vi "example_02_convert.vi"() -> ()   [LabVIEW 2015, in "lv-unit-conversion.lvlib"] (continued)
{"symbol"="bar/h", "name"="bar per hour", "dimension"="M/LT3", "is_si_unit"=TRUE, "category"="derived", "base_unit"="Pa/s", "conversion_reference"="DERIVED", "is_exact"=TRUE, "a"=0.0, "b"=100000.0, "c"=3600.0, "d"=0.0, "underlying_def"="", "description"=""}, {"symbol"="kPa/h", "name"="kilopascal per hour", "dimension"="M/LT3", "is_si_unit"=TRUE, "category"="derived", "base_unit"="Pa/s", "conversion_reference"="DERIVED", "is_exact"=TRUE, "a"=0.0, "b"=1000.0, "c"=3600.0, "d"=0.0, "underlying_def"="", "description"=""}, {"symbol"="kPa/min", "name"="kilopascal per min", "dimension"="M/LT3", "is_si_unit"=TRUE, "category"="derived", "base_unit"="Pa/s", "conversion_reference"="DERIVED", "is_exact"=TRUE, "a"=0.0, "b"=1000.0, "c"=60.0, "d"=0.0, "underlying_def"="", "description"=""}, {"symbol"="MPa/h", "name"="megapascal per hour", "dimension"="M/LT3", "is_si_unit"=TRUE, "category"="derived", "base_unit"="Pa/s", "conversion_reference"="DERIVED", "is_exact"=TRUE, "a"=0.0, "b"=1000000.0, "c"=3600.0, "d"=0.0, "underlying_def"="", "description"=""}, {"symbol"="Pa/h", "name"="pascal per hour", "dimension"="M/LT3", "is_si_unit"=TRUE, "category"="derived", "base_unit"="Pa/s", "conversion_reference"="DERIVED", "is_exact"=TRUE, "a"=0.0, "b"=1.0, "c"=3600.0, "d"=0.0, "underlying_def"="", "description"=""}, {"symbol"="psi/h", "name"="psi per hour", "dimension"="M/LT3", "is_si_unit"=TRUE, "category"="derived", "base_unit"="Pa/s", "conversion_reference"="DERIVED", "is_exact"=TRUE, "a"=0.0, "b"=4.4482216152605, "c"=2.322576, "d"=0.0, "underlying_def"="", "description"=""}, {"symbol"="psi/min", "name"="psi per minute", "dimension"="M/LT3", "is_si_unit"=TRUE, "category"="derived", "base_unit"="Pa/s", "conversion_reference"="DERIVED", "is_exact"=TRUE, "a"=0.0, "b"=4.4482216152605, "c"=0.0387096, "d"=0.0, "underlying_def"="", "description"=""}, {"symbol"="0.001 kPa2/cP", "name"="kilopascal squared per thousand centipoise", "dimension"="M/LT3", "is_si_unit"=TRUE, "category"="derived", "base_unit"="Pa2/(Pa.s)", "conversion_reference"="DERIVED", "is_exact"=TRUE, "a"=0.0, "b"=1000000.0, "c"=1.0, "d"=0.0, "underlying_def"="", "description"=""}, {"symbol"="bar2/cP", "name"="bar squared per centipoise", "dimension"="M/LT3", "is_si_unit"=TRUE, "category"="derived", "base_unit"="Pa2/(Pa.s)", "conversion_reference"="DERIVED", "is_exact"=TRUE, "a"=0.0, "b"=10000000000000.0, "c"=1.0, "d"=0.0, "underlying_def"="", "description"=""}, {"symbol"="kPa2/cP", "name"="kilopascal squared per centipoise", "dimension"="M/LT3", "is_si_unit"=TRUE, "category"="derived", "base_unit"="Pa2/(Pa.s)", "conversion_reference"="DERIVED", "is_exact"=TRUE, "a"=0.0, "b"=1000000000.0, "c"=1.0, "d"=0.0, "underlying_def"="", "description"=""}, {"symbol"="psi2/cP", "name"="psi squared per centipoise", "dimension"="M/LT3", "is_si_unit"=TRUE, "category"="derived", "base_unit"="Pa2/(Pa.s)", "conversion_reference"="DERIVED", "is_exact"=TRUE, "a"=0.0, "b"=19.786675538470732, "c"=4.162314256e-10, "d"=0.0, "underlying_def"="", "description"=""}, {"symbol"="Btu[IT]/(h.ft3)", "name"="BTU per hour cubic foot", "dimension"="M/LT3", "is_si_unit"=TRUE, "category"="derived", "base_unit"="W/m3", "conversion_reference"="DERIVED", "is_exact"=TRUE, "a"=0.0, "b"=1055.05585262, "c"=101.9406477312, "d"=0.0, "underlying_def"="", "description"=""}, {"symbol"="Btu[IT]/(s.ft3)", "name"="(BTU per second) per cubic foot", "dimension"="M/LT3", "is_si_unit"=TRUE, "category"="derived", "base_unit"="W/m3", "conversion_reference"="DERIVED", "is_exact"=TRUE, "a"=0.0, "b"=1055.05585262, "c"=0.028316846592, "d"=0.0, "underlying_def"="", "description"=""}, {"symbol"="cal[th]/(h.cm3)", "name"="calorie per hour cubic centimetre", "dimension"="M/LT3", "is_si_unit"=TRUE, "category"="derived", "base_unit"="W/m3", "conversion_reference"="DERIVED", "is_exact"=TRUE, "a"=0.0, "b"=4.184, "c"=0.0036, "d"=0.0, "underlying_def"="", "description"=""}, {"symbol"="cal[th]/(s.cm3)", "name"="calorie per second cubic centimetre", "dimension"="M/LT3", "is_si_unit"=TRUE, "category"="derived", "base_unit"="W/m3", "conversion_reference"="DERIVED", "is_exact"=TRUE, "a"=0.0, "b"=4184000.0, "c"=1.0, "d"=0.0, "underlying_def"="", "description"=""}, {"symbol"="hp/ft3", "name"="horsepower per cubic foot", "dimension"="M/LT3", "is_si_unit"=TRUE, "category"="derived", "base_unit"="W/m3", "conversion_reference"="DERIVED", "is_exact"=TRUE, "a"=0.0, "b"=745.6998715822702, "c"=0.028316846592, "d"=0.0, "underlying_def"="", "description"=""}, {"symbol"="kW/m3", "name"="kilowatt per cubic metre", "dimension"="M/LT3", "is_si_unit"=TRUE, "category"="derived", "base_unit"="W/m3", "conversion_reference"="DERIVED", "is_exact"=TRUE, "a"=0.0, "b"=1000.0, "c"=1.0, "d"=0.0, "underlying_def"="", "description"=""}, {"symbol"="uW/m3", "name"="microwatt per cubic metre", "dimension"="M/LT3", "is_si_unit"=TRUE, "category"="derived", "base_unit"="W/m3", "conversion_reference"="DERIVED", "is_exact"=TRUE, "a"=0.0, "b"=1e-06, "c"=1.0, "d"=0.0, "underlying_def"="", "description"=""}, {"symbol"="kg/mol", "name"="kilogram per mole", "dimension"="M/N", "is_si_unit"=TRUE, "category"="derived", "base_unit"="", "conversion_reference"="", "is_exact"=FALSE, "a"=0.0, "b"=0.0, "c"=0.0, "d"=0.0, "underlying_def"="", "description"=""}, {"symbol"="g/mol", "name"="gram per mole", "dimension"="M/N", "is_si_unit"=TRUE, "category"="derived", "base_unit"="kg/mol", "conversion_reference"="DERIVED", "is_exact"=TRUE, "a"=0.0, "b"=0.001, "c"=1.0, "d"=0.0, "underlying_def"="", "description"=""}, {"symbol"="lbm/lbmol", "name"="pound-mass per pound-mole", "dimension"="M/N", "is_si_unit"=TRUE, "category"="derived", "base_unit"="kg/mol", "conversion_reference"="DERIVED", "is_exact"=TRUE, "a"=0.0, "b"=0.001, "c"=1.0, "d"=0.0, "underlying_def"="", "description"=""}, {"symbol"="W/(m2.sr)", "name"="watt per square metre steradian", "dimension"="M/ST3", "is_si_unit"=TRUE, "category"="derived", "base_unit"="", "conversion_reference"="", "is_exact"=FALSE, "a"=0.0, "b"=0.0, "c"=0.0, "d"=0.0, "underlying_def"="", "description"=""}, {"symbol"="kg/s", "name"="kilogram per second", "dimension"="M/T", "is_si_unit"=TRUE, "category"="derived", "base_unit"="", "conversion_reference"="", "is_exact"=FALSE, "a"=0.0, "b"=0.0, "c"=0.0, "d"=0.0, "underlying_def"="", "description"=""}, {"symbol"="1E6 lbm/a", "name"="million pound-mass per julian-year", "dimension"="M/T", "is_si_unit"=TRUE, "category"="derived", "base_unit"="kg/s", "conversion_reference"="DERIVED", "is_exact"=TRUE, "a"=0.0, "b"=453592.37, "c"=31557600.0, "d"=0.0, "underlying_def"="", "description"=""}, {"symbol"="g/s", "name"="gram per second", "dimension"="M/T", "is_si_unit"=TRUE, "category"="derived", "base_unit"="kg/s", "conversion_reference"="DERIVED", "is_exact"=TRUE, "a"=0.0, "b"=0.001, "c"=1.0, "d"=0.0, "underlying_def"="", "description"=""}, {"symbol"="kg/d", "name"="kilogram per day", "dimension"="M/T", "is_si_unit"=TRUE, "category"="derived", "base_unit"="kg/s", "conversion_reference"="DERIVED", "is_exact"=TRUE, "a"=0.0, "b"=1.0, "c"=86400.0, "d"=0.0, "underlying_def"="", "description"=""}, {"symbol"="kg/h", "name"="kilogram per hour", "dimension"="M/T", "is_si_unit"=TRUE, "category"="derived", "base_unit"="kg/s", "conversion_reference"="DERIVED", "is_exact"=TRUE, "a"=0.0, "b"=1.0, "c"=3600.0, "d"=0.0, "underlying_def"="", "description"=""}, {"symbol"="kg/min", "name"="kilogram per min", "dimension"="M/T", "is_si_unit"=TRUE, "category"="derived", "base_unit"="kg/s", "conversion_reference"="DERIVED", "is_exact"=TRUE, "a"=0.0, "b"=1.0, "c"=60.0, "d"=0.0, "underlying_def"="", "description"=""}, {"symbol"="lbm/d", "name"="pound-mass per day", "dimension"="M/T", "is_si_unit"=TRUE, "category"="derived", "base_unit"="kg/s", "conversion_reference"="DERIVED", "is_exact"=TRUE, "a"=0.0, "b"=0.45359237, "c"=86400.0, "d"=0.0, "underlying_def"="", "description"=""}, {"symbol"="lbm/h", "name"="pound-mass per hour", "dimension"="M/T", "is_si_unit"=TRUE, "category"="derived", "base_unit"="kg/s", "conversion_reference"="DERIVED", "is_exact"=TRUE, "a"=0.0, "b"=0.45359237, "c"=3600.0, "d"=0.0, "underlying_def"="", "description"=""}, {"symbol"="lbm/min", "name"="pound-mass per minute", "dimension"="M/T", "is_si_unit"=TRUE, "category"="derived", "base_unit"="kg/s", "conversion_reference"="DERIVED", "is_exact"=TRUE, "a"=0.0, "b"=0.45359237, "c"=60.0, "d"=0.0, "underlying_def"="", "description"=""}, {"symbol"="lbm/s", "name"="pound-mass per second", "dimension"="M/T", "is_si_unit"=TRUE, "category"="derived", "base_unit"="kg/s", "conversion_reference"="DERIVED", "is_exact"=TRUE, "a"=0.0, "b"=0.45359237, "c"=1.0, "d"=0.0, "underlying_def"="", "description"=""}, {"symbol"="Mg/a", "name"="megagram per julian-year", "dimension"="M/T", "is_si_unit"=TRUE, "category"="derived", "base_unit"="kg/s", "conversion_reference"="DERIVED", "is_exact"=TRUE, "a"=0.0, "b"=1000.0, "c"=31557600.0, "d"=0.0, "underlying_def"="", "description"=""}, {"symbol"="Mg/d", "name"="megagram per day", "dimension"="M/T", "is_si_unit"=TRUE, "category"="derived", "base_unit"="kg/s", "conversion_reference"="DERIVED", "is_exact"=TRUE, "a"=0.0, "b"=1000.0, "c"=86400.0, "d"=0.0, "underlying_def"="", "description"=""}, {"symbol"="Mg/h", "name"="megagram per hour", "dimension"="M/T", "is_si_unit"=TRUE, "category"="derived", "base_unit"="kg/s", "conversion_reference"="DERIVED", "is_exact"=TRUE, "a"=0.0, "b"=1000.0, "c"=3600.0, "d"=0.0, "underlying_def"="", "description"=""}, {"symbol"="Mg/min", "name"="megagram per minute", "dimension"="M/T", "is_si_unit"=TRUE, "category"="derived", "base_unit"="kg/s", "conversion_reference"="DERIVED", "is_exact"=TRUE, "a"=0.0, "b"=1000.0, "c"=60.0, "d"=0.0, "underlying_def"="", "description"=""}, {"symbol"="t/a", "name"="tonne per julian-year", "dimension"="M/T", "is_si_unit"=TRUE, "category"="derived", "base_unit"="kg/s", "conversion_reference"="DERIVED", "is_exact"=TRUE, "a"=0.0, "b"=1000.0, "c"=31557600.0, "d"=0.0, "underlying_def"="", "description"=""}, {"symbol"="t/d", "name"="tonne per day", "dimension"="M/T", "is_si_unit"=TRUE, "category"="derived", "base_unit"="kg/s", "conversion_reference"="DERIVED", "is_exact"=TRUE, "a"=0.0, "b"=1000.0, "c"=86400.0, "d"=0.0, "underlying_def"="", "description"=""}, {"symbol"="t/h", "name"="tonne per hour", "dimension"="M/T", "is_si_unit"=TRUE, "category"="derived", "base_unit"="kg/s", "conversion_reference"="DERIVED", "is_exact"=TRUE, "a"=0.0, "b"=1000.0, "c"=3600.0, "d"=0.0, "underlying_def"="", "description"=""}, {"symbol"="t/min", "name"="tonne per minute", "dimension"="M/T", "is_si_unit"=TRUE, "category"="derived", "base_unit"="kg/s", "conversion_reference"="DERIVED", "is_exact"=TRUE, "a"=0.0, "b"=1000.0, "c"=60.0, "d"=0.0, "underlying_def"="", "description"=""}, {"symbol"="ton[UK]/a", "name"="UK ton-mass per julian-year", "dimension"="M/T", "is_si_unit"=TRUE, "category"="derived", "base_unit"="kg/s", "conversion_reference"="DERIVED", "is_exact"=TRUE, "a"=0.0, "b"=1016.0469088, "c"=31557600.0, "d"=0.0, "underlying_def"="", "description"=""}, {"symbol"="ton[UK]/d", "name"="UK ton-mass per day", "dimension"="M/T", "is_si_unit"=TRUE, "category"="derived", "base_unit"="kg/s", "conversion_reference"="DERIVED", "is_exact"=TRUE, "a"=0.0, "b"=1016.0469088, "c"=86400.0, "d"=0.0, "underlying_def"="", "description"=""}, {"symbol"="ton[UK]/h", "name"="UK ton-mass per hour", "dimension"="M/T", "is_si_unit"=TRUE, "category"="derived", "base_unit"="kg/s", "conversion_reference"="DERIVED", "is_exact"=TRUE, "a"=0.0, "b"=1016.0469088, "c"=3600.0, "d"=0.0, "underlying_def"="", "description"=""}, {"symbol"="ton[UK]/min", "name"="UK ton-mass per minute", "dimension"="M/T", "is_si_unit"=TRUE, "category"="derived", "base_unit"="kg/s", "conversion_reference"="DERIVED", "is_exact"=TRUE, "a"=0.0, "b"=1016.0469088, "c"=60.0, "d"=0.0, "underlying_def"="", "description"=""}, {"symbol"="ton[US]/a", "name"="US ton-mass per julian-year", "dimension"="M/T", "is_si_unit"=TRUE, "category"="derived", "base_unit"="kg/s", "conversion_reference"="DERIVED", "is_exact"=TRUE, "a"=0.0, "b"=907.18474, "c"=31557600.0, "d"=0.0, "underlying_def"="", "description"=""}, {"symbol"="ton[US]/d", "name"="US ton-mass per day", "dimension"="M/T", "is_si_unit"=TRUE, "category"="derived", "base_unit"="kg/s", "conversion_reference"="DERIVED", "is_exact"=TRUE, "a"=0.0, "b"=907.18474, "c"=86400.0, "d"=0.0, "underlying_def"="", "description"=""}, {"symbol"="ton[US]/h", "name"="US ton-mass per hour", "dimension"="M/T", "is_si_unit"=TRUE, "category"="derived", "base_unit"="kg/s", "conversion_reference"="DERIVED", "is_exact"=TRUE, "a"=0.0, "b"=907.18474, "c"=3600.0, "d"=0.0, "underlying_def"="", "description"=""}, {"symbol"="ton[US]/min", "name"="US ton-mass per minute", "dimension"="M/T", "is_si_unit"=TRUE, "category"="derived", "base_unit"="kg/s", "conversion_reference"="DERIVED", "is_exact"=TRUE, "a"=0.0, "b"=907.18474, "c"=60.0, "d"=0.0, "underlying_def"="", "description"=""}, {"symbol"="J/m2", "name"="joule per square metre", "dimension"="M/T2", "is_si_unit"=TRUE, "category"="derived", "base_unit"="", "conversion_reference"="", "is_exact"=FALSE, "a"=0.0, "b"=0.0, "c"=0.0, "d"=0.0, "underlying_def"="N/m", "description"=""}, {"symbol"="N/m", "name"="newton per metre", "dimension"="M/T2", "is_si_unit"=TRUE, "category"="derived", "base_unit"="", "conversion_reference"="", "is_exact"=FALSE, "a"=0.0, "b"=0.0, "c"=0.0, "d"=0.0, "underlying_def"="", "description"=""}, {"symbol"="erg/cm2", "name"="erg per square centimetre", "dimension"="M/T2", "is_si_unit"=TRUE, "category"="derived", "base_unit"="J/m2", "conversion_reference"="DERIVED", "is_exact"=TRUE, "a"=0.0, "b"=0.001, "c"=1.0, "d"=0.0, "underlying_def"="", "description"=""}, {"symbol"="J/cm2", "name"="joule per square centimetre", "dimension"="M/T2", "is_si_unit"=TRUE, "category"="derived", "base_unit"="J/m2", "conversion_reference"="DERIVED", "is_exact"=TRUE, "a"=0.0, "b"=10000.0, "c"=1.0, "d"=0.0, "underlying_def"="", "description"=""}, {"symbol"="kgf.m/cm2", "name"="thousand gram-force metre per square centimetre", "dimension"="M/T2", "is_si_unit"=TRUE, "category"="derived", "base_unit"="J/m2", "conversion_reference"="DERIVED", "is_exact"=TRUE, "a"=0.0, "b"=98066.5, "c"=1.0, "d"=0.0, "underlying_def"="", "description"=""}, {"symbol"="lbf.ft/in2", "name"="foot pound-force per square inch", "dimension"="M/T2", "is_si_unit"=TRUE, "category"="derived", "base_unit"="J/m2", "conversion_reference"="DERIVED", "is_exact"=TRUE, "a"=0.0, "b"=1.3558179483314003, "c"=0.00064516, "d"=0.0, "underlying_def"="", "description"=""}, {"symbol"="mJ/cm2", "name"="millijoule per square centimetre", "dimension"="M/T2", "is_si_unit"=TRUE, "category"="derived", "base_unit"="J/m2", "conversion_reference"="DERIVED", "is_exact"=TRUE, "a"=0.0, "b"=10.0, "c"=1.0, "d"=0.0, "underlying_def"="", "description"=""}, {"symbol"="mJ/m2", "name"="millijoule per square metre", "dimension"="M/T2", "is_si_unit"=TRUE, "category"="derived", "base_unit"="J/m2", "conversion_reference"="DERIVED", "is_exact"=TRUE, "a"=0.0, "b"=0.001, "c"=1.0, "d"=0.0, "underlying_def"="", "description"=""}, {"symbol"="0.01 lbf/ft", "name"="pound-force per hundred foot", "dimension"="M/T2", "is_si_unit"=TRUE, "category"="derived", "base_unit"="N/m", "conversion_reference"="DERIVED", "is_exact"=TRUE, "a"=0.0, "b"=4.4482216152605, "c"=30.48, "d"=0.0, "underlying_def"="", "description"=""}, {"symbol"="1/30 lbf/m", "name"="pound-force per thirty metre", "dimension"="M/T2", "is_si_unit"=TRUE, "category"="derived", "base_unit"="N/m", "conversion_reference"="DERIVED", "is_exact"=TRUE, "a"=0.0, "b"=4.4482216152605, "c"=30.0, "d"=0.0, "underlying_def"="", "description"=""}, {"symbol"="1/30 N/m", "name"="newton per thirty metre", "dimension"="M/T2", "is_si_unit"=TRUE, "category"="derived", "base_unit"="N/m", "conversion_reference"="DERIVED", "is_exact"=TRUE, "a"=0.0, "b"=1.0, "c"=30.0, "d"=0.0, "underlying_def"="", "description"=""}, {"symbol"="dyne/cm", "name"="dyne per centimetre", "dimension"="M/T2", "is_si_unit"=TRUE, "category"="derived", "base_unit"="N/m", "conversion_reference"="DERIVED", "is_exact"=TRUE, "a"=0.0, "b"=0.001, "c"=1.0, "d"=0.0, "underlying_def"="", "description"=""}, {"symbol"="kgf/cm", "name"="thousand gram-force per centimetre", "dimension"="M/T2", "is_si_unit"=TRUE, "category"="derived", "base_unit"="N/m", "conversion_reference"="DERIVED", "is_exact"=TRUE, "a"=0.0, "b"=980.665, "c"=1.0, "d"=0.0, "underlying_def"="", "description"=""}, {"symbol"="kN/m", "name"="kilonewton per metre", "dimension"="M/T2", "is_si_unit"=TRUE, "category"="derived", "base_unit"="N/m", "conversion_reference"="DERIVED", "is_exact"=TRUE, "a"=0.0, "b"=1000.0, "c"=1.0, "d"=0.0, "underlying_def"="", "description"=""}, {"symbol"="lbf/ft", "name"="pound-force per foot", "dimension"="M/T2", "is_si_unit"=TRUE, "category"="derived", "base_unit"="N/m", "conversion_reference"="DERIVED", "is_exact"=TRUE, "a"=0.0, "b"=4.4482216152605, "c"=0.3048, "d"=0.0, "underlying_def"="", "description"=""}, {"symbol"="lbf/in", "name"="pound-force per inch", "dimension"="M/T2", "is_si_unit"=TRUE, "category"="derived", "base_unit"="N/m", "conversion_reference"="DERIVED", "is_exact"=TRUE, "a"=0.0, "b"=4.4482216152605, "c"=0.0254, "d"=0.0, "underlying_def"="", "description"=""}, {"symbol"="mN/km", "name"="millinewton per kilometre", "dimension"="M/T2", "is_si_unit"=TRUE, "category"="derived", "base_unit"="N/m", "conversion_reference"="DERIVED", "is_exact"=TRUE, "a"=0.0, "b"=1e-06, "c"=1.0, "d"=0.0, "underlying_def"="", "description"=""}, {"symbol"="mN/m", "name"="millinewton per metre", "dimension"="M/T2", "is_si_unit"=TRUE, "category"="derived", "base_unit"="N/m", "conversion_reference"="DERIVED", "is_exact"=TRUE, "a"=0.0, "b"=0.001, "c"=1.0, "d"=0.0, "underlying_def"="", "description"=""}, {"symbol"="pdl/cm", "name"="poundal per centimetre", "dimension"="M/T2", "is_si_unit"=TRUE, "category"="derived", "base_unit"="N/m", "conversion_reference"="DERIVED", "is_exact"=TRUE, "a"=0.0, "b"=0.138254954376, "c"=0.01, "d"=0.0, "underlying_def"="", "description"=""}, {"symbol"="tonf[UK]/ft", "name"="UK ton-force per foot", "dimension"="M/T2", "is_si_unit"=TRUE, "category"="derived", "base_unit"="N/m", "conversion_reference"="DERIVED", "is_exact"=TRUE, "a"=0.0, "b"=9964.01641818352, "c"=0.3048, "d"=0.0, "underlying_def"="", "description"=""}, {"symbol"="tonf[US]/ft", "name"="US ton-force per foot", "dimension"="M/T2", "is_si_unit"=TRUE, "category"="derived", "base_unit"="N/m", "conversion_reference"="DERIVED", "is_exact"=TRUE, "a"=0.0, "b"=8896.443230521, "c"=0.3048, "d"=0.0, "underlying_def"="", "description"=""}, {"symbol"="W/m2", "name"="watt per square metre", "dimension"="M/T3", "is_si_unit"=TRUE, "category"="derived", "base_unit"="", "conversion_reference"="", "is_exact"=FALSE, "a"=0.0, "b"=0.0, "c"=0.0, "d"=0.0, "underlying_def"="", "description"=""}, {"symbol"="Btu[IT]/(h.ft2)", "name"="(BTU per hour) per square foot", "dimension"="M/T3", "is_si_unit"=TRUE, "category"="derived", "base_unit"="W/m2", "conversion_reference"="DERIVED", "is_exact"=TRUE, "a"=0.0, "b"=1055.05585262, "c"=334.450944, "d"=0.0, "underlying_def"="", "description"=""}, {"symbol"="Btu[IT]/(s.ft2)", "name"="BTU per second square foot", "dimension"="M/T3", "is_si_unit"=TRUE, "category"="derived", "base_unit"="W/m2", "conversion_reference"="DERIVED", "is_exact"=TRUE, "a"=0.0, "b"=1055.05585262, "c"=0.09290304, "d"=0.0, "underlying_def"="", "description"=""}, {"symbol"="cal[th]/(h.cm2)", "name"="calorie per hour square centimetre", "dimension"="M/T3", "is_si_unit"=TRUE, "category"="derived", "base_unit"="W/m2", "conversion_reference"="DERIVED", "is_exact"=TRUE, "a"=0.0, "b"=4.184, "c"=0.36, "d"=0.0, "underlying_def"="", "description"=""}, {"symbol"="hp/in2", "name"="horsepower per square inch", "dimension"="M/T3", "is_si_unit"=TRUE, "category"="derived", "base_unit"="W/m2", "conversion_reference"="DERIVED", "is_exact"=TRUE, "a"=0.0, "b"=745.6998715822702, "c"=0.00064516, "d"=0.0, "underlying_def"="", "description"=""}, {"symbol"="hp[hyd]/in2", "name"="hydraulic-horsepower per square inch", "dimension"="M/T3", "is_si_unit"=TRUE, "category"="derived", "base_unit"="W/m2", "conversion_reference"="DERIVED", "is_exact"=TRUE, "a"=0.0, "b"=746.043, "c"=0.00064516, "d"=0.0, "underlying_def"="", "description"=""}, {"symbol"="kW/cm2", "name"="kilowatt per square centimetre", "dimension"="M/T3", "is_si_unit"=TRUE, "category"="derived", "base_unit"="W/m2", "conversion_reference"="DERIVED", "is_exact"=TRUE, "a"=0.0, "b"=10000000.0, "c"=1.0, "d"=0.0, "underlying_def"="", "description"=""}, {"symbol"="kW/m2", "name"="kilowatt per square metre", "dimension"="M/T3", "is_si_unit"=TRUE, "category"="derived", "base_unit"="W/m2", "conversion_reference"="DERIVED", "is_exact"=TRUE, "a"=0.0, "b"=1000.0, "c"=1.0, "d"=0.0, "underlying_def"="", "description"=""}, {"symbol"="mW/m2", "name"="milliwatt per square metre", "dimension"="M/T3", "is_si_unit"=TRUE, "category"="derived", "base_unit"="W/m2", "conversion_reference"="DERIVED", "is_exact"=TRUE, "a"=0.0, "b"=0.001, "c"=1.0, "d"=0.0, "underlying_def"="", "description"=""}, {"symbol"="ucal[th]/(s.cm2)", "name"="millionth of calorie per second square centimetre", "dimension"="M/T3", "is_si_unit"=TRUE, "category"="derived", "base_unit"="W/m2", "conversion_reference"="DERIVED", "is_exact"=TRUE, "a"=0.0, "b"=0.04184, "c"=1.0, "d"=0.0, "underlying_def"="", "description"=""}, {"symbol"="W/cm2", "name"="watt per square centimetre", "dimension"="M/T3", "is_si_unit"=TRUE, "category"="derived", "base_unit"="W/m2", "conversion_reference"="DERIVED", "is_exact"=TRUE, "a"=0.0, "b"=10000.0, "c"=1.0, "d"=0.0, "underlying_def"="", "description"=""}, {"symbol"="W/mm2", "name"="watt per square millimetre", "dimension"="M/T3", "is_si_unit"=TRUE, "category"="derived", "base_unit"="W/m2", "conversion_reference"="DERIVED", "is_exact"=TRUE, "a"=0.0, "b"=1000000.0, "c"=1.0, "d"=0.0, "underlying_def"="", "description"=""}, {"symbol"="GPa2", "name"="gigapascal squared", "dimension"="M2/L2T4", "is_si_unit"=TRUE, "category"="derived", "base_unit"="Pa2", "conversion_reference"="DERIVED", "is_exact"=TRUE, "a"=0.0, "b"=1e+18, "c"=1.0, "d"=0.0, "underlying_def"="", "description"=""}, {"symbol"="kPa2", "name"="kilopascal squared", "dimension"="M2/L2T4", "is_si_unit"=TRUE, "category"="derived", "base_unit"="Pa2", "conversion_reference"="DERIVED", "is_exact"=TRUE, "a"=0.0, "b"=1000000.0, "c"=1.0, "d"=0.0, "underlying_def"="", "description"=""}, {"symbol"="kpsi2", "name"="(thousand psi) squared", "dimension"="M2/L2T4", "is_si_unit"=TRUE, "category"="derived", "base_unit"="Pa2", "conversion_reference"="DERIVED", "is_exact"=TRUE, "a"=0.0, "b"=19786675.53847073, "c"=4.162314256e-07, "d"=0.0, "underlying_def"="", "description"=""}, {"symbol"="Pa2", "name"="pascal squared", "dimension"="M2/L2T4", "is_si_unit"=TRUE, "category"="derived", "base_unit"="", "conversion_reference"="", "is_exact"=FALSE, "a"=0.0, "b"=0.0, "c"=0.0, "d"=0.0, "underlying_def"="", "description"=""}, {"symbol"="bar2", "name"="bar squared", "dimension"="M2/L2T4", "is_si_unit"=TRUE, "category"="derived", "base_unit"="Pa2", "conversion_reference"="DERIVED", "is_exact"=TRUE, "a"=0.0, "b"=10000000000.0, "c"=1.0, "d"=0.0, "underlying_def"="", "description"=""}, {"symbol"="psi2", "name"="psi squared", "dimension"="M2/L2T4", "is_si_unit"=TRUE, "category"="derived", "base_unit"="Pa2", "conversion_reference"="DERIVED", "is_exact"=TRUE, "a"=0.0, "b"=19.786675538470732, "c"=4.162314256e-07, "d"=0.0, "underlying_def"="", "description"=""}, {"symbol"="mol", "name"="gram-mole", "dimension"="N", "is_si_unit"=TRUE, "category"="atom-base", "base_unit"="", "conversion_reference"="", "is_exact"=FALSE, "a"=0.0, "b"=0.0, "c"=0.0, "d"=0.0, "underlying_def"="", "description"="The mole is the amount (in grams) of substance of a system that contains as many elementary entities \n\t\t\t\tas there are atoms in 0.012 kilogram of carbon-12. \n\t\t\t\tWhen the mole is used, the elementary entities must be specified and may be atoms, molecules, ions, \n\t\t\t\telectrons, other particles, or specified groups of such particles.\n\t\t\t"}, {"symbol"="lbmol", "name"="pound-mass-mole", "dimension"="N", "is_si_unit"=TRUE, "category"="atom", "base_unit"="mol", "conversion_reference"="DEFINITION", "is_exact"=TRUE, "a"=0.0, "b"=453.59237, "c"=1.0, "d"=0.0, "underlying_def"="", "description"="The amount (in pound-mass) of substance of a system which contains as many elementary entities as \n\t\t\t\tthere are atoms in 0.012 kilogram of carbon 12. \n\t\t\t\tThe conversion involves converting pound-mass to kilograms.\n\t\t\t"}, {"symbol"="kmol", "name"="kilogram-mole", "dimension"="N", "is_si_unit"=TRUE, "category"="prefixed", "base_unit"="mol", "conversion_reference"="DERIVED", "is_exact"=TRUE, "a"=0.0, "b"=1000.0, "c"=1.0, "d"=0.0, "underlying_def"="", "description"=""}, {"symbol"="mmol", "name"="milligram-mole", "dimension"="N", "is_si_unit"=TRUE, "category"="prefixed", "base_unit"="mol", "conversion_reference"="DERIVED", "is_exact"=TRUE, "a"=0.0, "b"=0.001, "c"=1.0, "d"=0.0, "underlying_def"="", "description"=""}, {"symbol"="umol", "name"="microgram-mole", "dimension"="N", "is_si_unit"=TRUE, "category"="prefixed", "base_unit"="mol", "conversion_reference"="DERIVED", "is_exact"=TRUE, "a"=0.0, "b"=1e-06, "c"=1.0, "d"=0.0, "underlying_def"="", "description"=""}, {"symbol"="mol/m2", "name"="gram-mole per square metre", "dimension"="N/L2", "is_si_unit"=TRUE, "category"="derived", "base_unit"="", "conversion_reference"="", "is_exact"=FALSE, "a"=0.0, "b"=0.0, "c"=0.0, "d"=0.0, "underlying_def"="", "description"=""}, {"symbol"="mol/(s.m2)", "name"="gram-mole per second square metre", "dimension"="N/L2T", "is_si_unit"=TRUE, "category"="derived", "base_unit"="", "conversion_reference"="", "is_exact"=FALSE, "a"=0.0, "b"=0.0, "c"=0.0, "d"=0.0, "underlying_def"="", "description"=""}, {"symbol"="lbmol/(h.ft2)", "name"="pound-mass-mole per hour square foot", "dimension"="N/L2T", "is_si_unit"=TRUE, "category"="derived", "base_unit"="mol/(s.m2)", "conversion_reference"="DERIVED", "is_exact"=TRUE, "a"=0.0, "b"=453.59237, "c"=334.450944, "d"=0.0, "underlying_def"="", "description"=""}, {"symbol"="lbmol/(s.ft2)", "name"="pound-mass-mole per second square foot", "dimension"="N/L2T", "is_si_unit"=TRUE, "category"="derived", "base_unit"="mol/(s.m2)", "conversion_reference"="DERIVED", "is_exact"=TRUE, "a"=0.0, "b"=453.59237, "c"=0.09290304, "d"=0.0, "underlying_def"="", "description"=""}, {"symbol"="mol/m3", "name"="gram-mole per cubic metre", "dimension"="N/L3", "is_si_unit"=TRUE, "category"="derived", "base_unit"="", "conversion_reference"="", "is_exact"=FALSE, "a"=0.0, "b"=0.0, "c"=0.0, "d"=0.0, "underlying_def"="", "description"=""}, {"symbol"="kmol/m3", "name"="kilogram-mole per cubic metre", "dimension"="N/L3", "is_si_unit"=TRUE, "category"="derived", "base_unit"="mol/m3", "conversion_reference"="DERIVED", "is_exact"=TRUE, "a"=0.0, "b"=1000.0, "c"=1.0, "d"=0.0, "underlying_def"="", "description"=""}, {"symbol"="lbmol/ft3", "name"="pound-mass-mole per cubic foot", "dimension"="N/L3", "is_si_unit"=TRUE, "category"="derived", "base_unit"="mol/m3", "conversion_reference"="DERIVED", "is_exact"=TRUE, "a"=0.0, "b"=453.59237, "c"=0.028316846592, "d"=0.0, "underlying_def"="", "description"=""}, {"symbol"="lbmol/gal[UK]", "name"="pound-mass-mole per UK gallon", "dimension"="N/L3", "is_si_unit"=TRUE, "category"="derived", "base_unit"="mol/m3", "conversion_reference"="DERIVED", "is_exact"=TRUE, "a"=0.0, "b"=453.59237, "c"=0.00454609, "d"=0.0, "underlying_def"="", "description"=""}, {"symbol"="lbmol/gal[US]", "name"="pound-mass-mole per US gallon", "dimension"="N/L3", "is_si_unit"=TRUE, "category"="derived", "base_unit"="mol/m3", "conversion_reference"="DERIVED", "is_exact"=TRUE, "a"=0.0, "b"=453.59237, "c"=0.003785411784, "d"=0.0, "underlying_def"="", "description"=""}, {"symbol"="mol/s", "name"="gram-mole per second", "dimension"="N/T", "is_si_unit"=TRUE, "category"="derived", "base_unit"="", "conversion_reference"="", "is_exact"=FALSE, "a"=0.0, "b"=0.0, "c"=0.0, "d"=0.0, "underlying_def"="", "description"=""}, {"symbol"="kmol/h", "name"="kilogram-mole per hour", "dimension"="N/T", "is_si_unit"=TRUE, "category"="derived", "base_unit"="mol/s", "conversion_reference"="DERIVED", "is_exact"=TRUE, "a"=0.0, "b"=1000.0, "c"=3600.0, "d"=0.0, "underlying_def"="", "description"=""}, {"symbol"="kmol/s", "name"="kilogram-mole per second", "dimension"="N/T", "is_si_unit"=TRUE, "category"="derived", "base_unit"="mol/s", "conversion_reference"="DERIVED", "is_exact"=TRUE, "a"=0.0, "b"=1000.0, "c"=1.0, "d"=0.0, "underlying_def"="", "description"=""}, {"symbol"="lbmol/h", "name"="pound-mass-mole per hour", "dimension"="N/T", "is_si_unit"=TRUE, "category"="derived", "base_unit"="mol/s", "conversion_reference"="DERIVED", "is_exact"=TRUE, "a"=0.0, "b"=453.59237, "c"=3600.0, "d"=0.0, "underlying_def"="", "description"=""}, {"symbol"="lbmol/s", "name"="pound-mass-mole per second", "dimension"="N/T", "is_si_unit"=TRUE, "category"="derived", "base_unit"="mol/s", "conversion_reference"="DERIVED", "is_exact"=TRUE, "a"=0.0, "b"=453.59237, "c"=1.0, "d"=0.0, "underlying_def"="", "description"=""}, {"symbol"="sr", "name"="steradian", "dimension"="S", "is_si_unit"=TRUE, "category"="atom-special", "base_unit"="", "conversion_reference"="", "is_exact"=FALSE, "a"=0.0, "b"=0.0, "c"=0.0, "d"=0.0, "underlying_def"="", "description"="The steradian is the solid angle that, having its vertex in the center of a circle, cuts of an area \n\t\t\t\tof the surface of the sphere equal to that of a square with sides of length equal to the radius of \n\t\t\t\tthe sphere.\n\t\t\t"}, {"symbol"="s", "name"="second", "dimension"="T", "is_si_unit"=TRUE, "category"="atom-base", "base_unit"="", "conversion_reference"="", "is_exact"=FALSE, "a"=0.0, "b"=0.0, "c"=0.0, "d"=0.0, "underlying_def"="", "description"="The second is the duration of 9 192 631 770 periods of the radiation corresponding to the transition \n\t\t\t\tbetween the two hyperfine levels of the ground state of the cesium-133 atom.\n\t\t\t"}, {"symbol"="a", "name"="julian-year", "dimension"="T", "is_si_unit"=TRUE, "category"="atom", "base_unit"="s", "conversion_reference"="DEFINITION", "is_exact"=TRUE, "a"=0.0, "b"=31557600.0, "c"=1.0, "d"=0.0, "underlying_def"="365.25 d", "description"="The underlying definition taken from NIST statement that \"Julian century = 36 525 d\"."}, {"symbol"="a[t]", "name"="tropical-year", "dimension"="T", "is_si_unit"=TRUE, "category"="atom", "base_unit"="s", "conversion_reference"="IUGS-year", "is_exact"=TRUE, "a"=0.0, "b"=31556925.445, "c"=1.0, "d"=0.0, "underlying_def"="", "description"="The year as a defined multiple of the second that minimizes time-dependent inaccuracy. \n\t\t\t\tUsed for expressing very long time intervals both for earth scientists and nuclear physicists alike. \n\t\t\t\tTakes into account the non-relativistic estimate of astronomical decrease by 0.530 s per century, \n\t\t\t\tfor the epoch 2000.0. \n\t\t\t\tFrom \"International Union of Geological Sciences\" (IUPAC Recommendation 2011).\n\t\t\t"}, {"symbol"="d", "name"="day", "dimension"="T", "is_si_unit"=TRUE, "category"="atom-allowed", "base_unit"="s", "conversion_reference"="NIST-SI", "is_exact"=TRUE, "a"=0.0, "b"=86400.0, "c"=1.0, "d"=0.0, "underlying_def"="24 h", "description"="24 hours."}, {"symbol"="h", "name"="hour", "dimension"="T", "is_si_unit"=TRUE, "category"="atom-allowed", "base_unit"="s", "conversion_reference"="NIST-SI", "is_exact"=TRUE, "a"=0.0, "b"=3600.0, "c"=1.0, "d"=0.0, "underlying_def"="60 min", "description"="One twenty-fourth of a day or 60 minutes."}, {"symbol"="min", "name"="minute", "dimension"="T", "is_si_unit"=TRUE, "category"="atom-allowed", "base_unit"="s", "conversion_reference"="NIST-SI", "is_exact"=TRUE, "a"=0.0, "b"=60.0, "c"=1.0, "d"=0.0, "underlying_def"="60 s", "description"="60 seconds."}, {"symbol"="wk", "name"="week", "dimension"="T", "is_si_unit"=TRUE, "category"="atom", "base_unit"="s", "conversion_reference"="DEFINITION", "is_exact"=TRUE, "a"=0.0, "b"=604800.0, "c"=1.0, "d"=0.0, "underlying_def"="7 d", "description"="A week is seven days."}, {"symbol"="1/2 ms", "name"="half of millisecond", "dimension"="T", "is_si_unit"=TRUE, "category"="derived", "base_unit"="s", "conversion_reference"="DERIVED", "is_exact"=TRUE, "a"=0.0, "b"=0.0005, "c"=1.0, "d"=0.0, "underlying_def"="", "description"=""}, {"symbol"="100 ka[t]", "name"="hundred thousand tropical-year", "dimension"="T", "is_si_unit"=TRUE, "category"="derived", "base_unit"="s", "conversion_reference"="DERIVED", "is_exact"=TRUE, "a"=0.0, "b"=3155692544500.0, "c"=1.0, "d"=0.0, "underlying_def"="", "description"=""}, {"symbol"="ca", "name"="hundredth of julian-year", "dimension"="T", "is_si_unit"=TRUE, "category"="prefixed", "base_unit"="s", "conversion_reference"="DERIVED", "is_exact"=TRUE, "a"=0.0, "b"=315576.0, "c"=1.0, "d"=0.0, "underlying_def"="", "description"=""}, {"symbol"="cs", "name"="centisecond", "dimension"="T", "is_si_unit"=TRUE, "category"="prefixed", "base_unit"="s", "conversion_reference"="DERIVED", "is_exact"=TRUE, "a"=0.0, "b"=0.01, "c"=1.0, "d"=0.0, "underlying_def"="", "description"=""}, {"symbol"="ds", "name"="decisecond", "dimension"="T", "is_si_unit"=TRUE, "category"="prefixed", "base_unit"="s", "conversion_reference"="DERIVED", "is_exact"=TRUE, "a"=0.0, "b"=0.1, "c"=1.0, "d"=0.0, "underlying_def"="", "description"=""}, {"symbol"="Ea[t]", "name"="million million million tropical-year", "dimension"="T", "is_si_unit"=TRUE, "category"="prefixed", "base_unit"="s", "conversion_reference"="DERIVED", "is_exact"=TRUE, "a"=0.0, "b"=3.1556925445e+25, "c"=1.0, "d"=0.0, "underlying_def"="", "description"=""}, {"symbol"="fa", "name"="femtojulian-year", "dimension"="T", "is_si_unit"=TRUE, "category"="prefixed", "base_unit"="s", "conversion_reference"="DERIVED", "is_exact"=TRUE, "a"=0.0, "b"=3.15576e-08, "c"=1.0, "d"=0.0, "underlying_def"="", "description"=""}, {"symbol"="Ga[t]", "name"="thousand million tropical-year", "dimension"="T", "is_si_unit"=TRUE, "category"="prefixed", "base_unit"="s", "conversion_reference"="DERIVED", "is_exact"=TRUE, "a"=0.0, "b"=3.1556925445e+16, "c"=1.0, "d"=0.0, "underlying_def"="", "description"=""}, {"symbol"="hs", "name"="hectosecond", "dimension"="T", "is_si_unit"=TRUE, "category"="prefixed", "base_unit"="s", "conversion_reference"="DERIVED", "is_exact"=TRUE, "a"=0.0, "b"=100.0, "c"=1.0, "d"=0.0, "underlying_def"="", "description"=""}, {"symbol"="ka[t]", "name"="thousand tropical-year", "dimension"="T", "is_si_unit"=TRUE, "category"="prefixed", "base_unit"="s", "conversion_reference"="DERIVED", "is_exact"=TRUE, "a"=0.0, "b"=31556925445.0, "c"=1.0, "d"=0.0, "underlying_def"="", "description"=""}, {"symbol"="Ma[t]", "name"="million tropical-year", "dimension"="T", "is_si_unit"=TRUE, "category"="prefixed", "base_unit"="s", "conversion_reference"="DERIVED", "is_exact"=TRUE, "a"=0.0, "b"=31556925445000.0, "c"=1.0, "d"=0.0, "underlying_def"="", "description"=""}, {"symbol"="ms", "name"="millisecond", "dimension"="T", "is_si_unit"=TRUE, "category"="prefixed", "base_unit"="s", "conversion_reference"="DERIVED", "is_exact"=TRUE, "a"=0.0, "b"=0.001, "c"=1.0, "d"=0.0, "underlying_def"="", "description"=""}, {"symbol"="na", "name"="nanojulian-year", "dimension"="T", "is_si_unit"=TRUE, "category"="prefixed", "base_unit"="s", "conversion_reference"="DERIVED", "is_exact"=TRUE, "a"=0.0, "b"=0.0315576, "c"=1.0, "d"=0.0, "underlying_def"="", "description"=""}, {"symbol"="ns", "name"="nanosecond", "dimension"="T", "is_si_unit"=TRUE, "category"="prefixed", "base_unit"="s", "conversion_reference"="DERIVED", "is_exact"=TRUE, "a"=0.0, "b"=1e-09, "c"=1.0, "d"=0.0, "underlying_def"="", "description"=""}, {"symbol"="ps", "name"="picosecond", "dimension"="T", "is_si_unit"=TRUE, "category"="prefixed", "base_unit"="s", "conversion_reference"="DERIVED", "is_exact"=TRUE, "a"=0.0, "b"=1e-12, "c"=1.0, "d"=0.0, "underlying_def"="", "description"=""}, {"symbol"="Ta[t]", "name"="million million tropical-year", "dimension"="T", "is_si_unit"=TRUE, "category"="prefixed", "base_unit"="s", "conversion_reference"="DERIVED", "is_exact"=TRUE, "a"=0.0, "b"=3.1556925445e+19, "c"=1.0, "d"=0.0, "underlying_def"="", "description"=""}, {"symbol"="us", "name"="microsecond", "dimension"="T", "is_si_unit"=TRUE, "category"="prefixed", "base_unit"="s", "conversion_reference"="DERIVED", "is_exact"=TRUE, "a"=0.0, "b"=1e-06, "c"=1.0, "d"=0.0, "underlying_def"="", "description"=""}, {"symbol"="s/m", "name"="second per metre", "dimension"="T/L", "is_si_unit"=TRUE, "category"="derived", "base_unit"="", "conversion_reference"="", "is_exact"=FALSE, "a"=0.0, "b"=0.0, "c"=0.0, "d"=0.0, "underlying_def"="", "description"=""}, {"symbol"="0.001 h/ft", "name"="hour per thousand foot", "dimension"="T/L", "is_si_unit"=TRUE, "category"="derived", "base_unit"="s/m", "conversion_reference"="DERIVED", "is_exact"=TRUE, "a"=0.0, "b"=3600.0, "c"=304.8, "d"=0.0, "underlying_def"="", "description"=""}, {"symbol"="h/km", "name"="hour per kilometre", "dimension"="T/L", "is_si_unit"=TRUE, "category"="derived", "base_unit"="s/m", "conversion_reference"="DERIVED", "is_exact"=TRUE, "a"=0.0, "b"=3.6, "c"=1.0, "d"=0.0, "underlying_def"="", "description"=""}, {"symbol"="min/ft", "name"="minute per foot", "dimension"="T/L", "is_si_unit"=TRUE, "category"="derived", "base_unit"="s/m", "conversion_reference"="DERIVED", "is_exact"=TRUE, "a"=0.0, "b"=60.0, "c"=0.3048, "d"=0.0, "underlying_def"="", "description"=""}, {"symbol"="min/m", "name"="minute per metre", "dimension"="T/L", "is_si_unit"=TRUE, "category"="derived", "base_unit"="s/m", "conversion_reference"="DERIVED", "is_exact"=TRUE, "a"=0.0, "b"=60.0, "c"=1.0, "d"=0.0, "underlying_def"="", "description"=""}, {"symbol"="ms/cm", "name"="millisecond per centimetre", "dimension"="T/L", "is_si_unit"=TRUE, "category"="derived", "base_unit"="s/m", "conversion_reference"="DERIVED", "is_exact"=TRUE, "a"=0.0, "b"=0.1, "c"=1.0, "d"=0.0, "underlying_def"="", "description"=""}, {"symbol"="ms/ft", "name"="millisecond per foot", "dimension"="T/L", "is_si_unit"=TRUE, "category"="derived", "base_unit"="s/m", "conversion_reference"="DERIVED", "is_exact"=TRUE, "a"=0.0, "b"=0.001, "c"=0.3048, "d"=0.0, "underlying_def"="", "description"=""}, {"symbol"="ms/in", "name"="millisecond per inch", "dimension"="T/L", "is_si_unit"=TRUE, "category"="derived", "base_unit"="s/m", "conversion_reference"="DERIVED", "is_exact"=TRUE, "a"=0.0, "b"=0.001, "c"=0.0254, "d"=0.0, "underlying_def"="", "description"=""}, {"symbol"="ms/m", "name"="millisecond per metre", "dimension"="T/L", "is_si_unit"=TRUE, "category"="derived", "base_unit"="s/m", "conversion_reference"="DERIVED", "is_exact"=TRUE, "a"=0.0, "b"=0.001, "c"=1.0, "d"=0.0, "underlying_def"="", "description"=""}, {"symbol"="ns/ft", "name"="nanosecond per foot", "dimension"="T/L", "is_si_unit"=TRUE, "category"="derived", "base_unit"="s/m", "conversion_reference"="DERIVED", "is_exact"=TRUE, "a"=0.0, "b"=1e-09, "c"=0.3048, "d"=0.0, "underlying_def"="", "description"=""}, {"symbol"="ns/m", "name"="nanosecond per metre", "dimension"="T/L", "is_si_unit"=TRUE, "category"="derived", "base_unit"="s/m", "conversion_reference"="DERIVED", "is_exact"=TRUE, "a"=0.0, "b"=1e-09, "c"=1.0, "d"=0.0, "underlying_def"="", "description"=""}, {"symbol"="s/cm", "name"="second per centimetre", "dimension"="T/L", "is_si_unit"=TRUE, "category"="derived", "base_unit"="s/m", "conversion_reference"="DERIVED", "is_exact"=TRUE, "a"=0.0, "b"=100.0, "c"=1.0, "d"=0.0, "underlying_def"="", "description"=""}, {"symbol"="s/ft", "name"="second per foot", "dimension"="T/L", "is_si_unit"=TRUE, "category"="derived", "base_unit"="s/m", "conversion_reference"="DERIVED", "is_exact"=TRUE, "a"=0.0, "b"=1.0, "c"=0.3048, "d"=0.0, "underlying_def"="", "description"=""}, {"symbol"="s/in", "name"="second per inch", "dimension"="T/L", "is_si_unit"=TRUE, "category"="derived", "base_unit"="s/m", "conversion_reference"="DERIVED", "is_exact"=TRUE, "a"=0.0, "b"=1.0, "c"=0.0254, "d"=0.0, "underlying_def"="", "description"=""}, {"symbol"="us/ft", "name"="microsecond per foot", "dimension"="T/L", "is_si_unit"=TRUE, "category"="derived", "base_unit"="s/m", "conversion_reference"="DERIVED", "is_exact"=TRUE, "a"=0.0, "b"=1e-06, "c"=0.3048, "d"=0.0, "underlying_def"="", "description"=""}, {"symbol"="us/in", "name"="microsecond per inch", "dimension"="T/L", "is_si_unit"=TRUE, "category"="derived", "base_unit"="s/m", "conversion_reference"="DERIVED", "is_exact"=TRUE, "a"=0.0, "b"=1e-06, "c"=0.0254, "d"=0.0, "underlying_def"="", "description"=""}, {"symbol"="us/m", "name"="microsecond per metre", "dimension"="T/L", "is_si_unit"=TRUE, "category"="derived", "base_unit"="s/m", "conversion_reference"="DERIVED", "is_exact"=TRUE, "a"=0.0, "b"=1e-06, "c"=1.0, "d"=0.0, "underlying_def"="", "description"=""}, {"symbol"="s/m3", "name"="second per cubic metre", "dimension"="T/L3", "is_si_unit"=TRUE, "category"="derived", "base_unit"="", "conversion_reference"="", "is_exact"=FALSE, "a"=0.0, "b"=0.0, "c"=0.0, "d"=0.0, "underlying_def"="", "description"=""}, {"symbol"="0.001 d/ft3", "name"="day per thousand cubic foot", "dimension"="T/L3", "is_si_unit"=TRUE, "category"="derived", "base_unit"="s/m3", "conversion_reference"="DERIVED", "is_exact"=TRUE, "a"=0.0, "b"=86400.0, "c"=28.316846592, "d"=0.0, "underlying_def"="", "description"=""}, {"symbol"="d/bbl", "name"="day per barrel", "dimension"="T/L3", "is_si_unit"=TRUE, "category"="derived", "base_unit"="s/m3", "conversion_reference"="DERIVED", "is_exact"=TRUE, "a"=0.0, "b"=86400.0, "c"=0.158987294928, "d"=0.0, "underlying_def"="", "description"=""}, {"symbol"="d/ft3", "name"="day per cubic foot", "dimension"="T/L3", "is_si_unit"=TRUE, "category"="derived", "base_unit"="s/m3", "conversion_reference"="DERIVED", "is_exact"=TRUE, "a"=0.0, "b"=86400.0, "c"=0.028316846592, "d"=0.0, "underlying_def"="", "description"=""}, {"symbol"="d/m3", "name"="day per cubic metre", "dimension"="T/L3", "is_si_unit"=TRUE, "category"="derived", "base_unit"="s/m3", "conversion_reference"="DERIVED", "is_exact"=TRUE, "a"=0.0, "b"=86400.0, "c"=1.0, "d"=0.0, "underlying_def"="", "description"=""}, {"symbol"="h/ft3", "name"="hour per cubic foot", "dimension"="T/L3", "is_si_unit"=TRUE, "category"="derived", "base_unit"="s/m3", "conversion_reference"="DERIVED", "is_exact"=TRUE, "a"=0.0, "b"=3600.0, "c"=0.028316846592, "d"=0.0, "underlying_def"="", "description"=""}, {"symbol"="h/m3", "name"="hour per cubic metre", "dimension"="T/L3", "is_si_unit"=TRUE, "category"="derived", "base_unit"="s/m3", "conversion_reference"="DERIVED", "is_exact"=TRUE, "a"=0.0, "b"=3600.0, "c"=1.0, "d"=0.0, "underlying_def"="", "description"=""}, {"symbol"="s/ft3", "name"="second per cubic foot", "dimension"="T/L3", "is_si_unit"=TRUE, "category"="derived", "base_unit"="s/m3", "conversion_reference"="DERIVED", "is_exact"=TRUE, "a"=0.0, "b"=1.0, "c"=0.028316846592, "d"=0.0, "underlying_def"="", "description"=""}, {"symbol"="s/L", "name"="second per litre", "dimension"="T/L3", "is_si_unit"=TRUE, "category"="derived", "base_unit"="s/m3", "conversion_reference"="DERIVED", "is_exact"=TRUE, "a"=0.0, "b"=1000.0, "c"=1.0, "d"=0.0, "underlying_def"="", "description"=""}, {"symbol"="s/qt[UK]", "name"="second per UK quart", "dimension"="T/L3", "is_si_unit"=TRUE, "category"="derived", "base_unit"="s/m3", "conversion_reference"="DERIVED", "is_exact"=TRUE, "a"=0.0, "b"=1.0, "c"=0.0011365225, "d"=0.0, "underlying_def"="", "description"=""}, {"symbol"="s/qt[US]", "name"="second per US quart", "dimension"="T/L3", "is_si_unit"=TRUE, "category"="derived", "base_unit"="s/m3", "conversion_reference"="DERIVED", "is_exact"=TRUE, "a"=0.0, "b"=1.0, "c"=0.000946352946, "d"=0.0, "underlying_def"="", "description"=""}, {"symbol"="s/kg", "name"="second per kilogram", "dimension"="T/M", "is_si_unit"=TRUE, "category"="derived", "base_unit"="", "conversion_reference"="", "is_exact"=FALSE, "a"=0.0, "b"=0.0, "c"=0.0, "d"=0.0, "underlying_def"="", "description"=""}, {"symbol"="kg/J", "name"="kilogram per joule", "dimension"="T2/L2", "is_si_unit"=TRUE, "category"="derived", "base_unit"="", "conversion_reference"="", "is_exact"=FALSE, "a"=0.0, "b"=0.0, "c"=0.0, "d"=0.0, "underlying_def"="", "description"=""}, {"symbol"="kg/(kW.h)", "name"="kilogram per kilowatt hour", "dimension"="T2/L2", "is_si_unit"=TRUE, "category"="derived", "base_unit"="kg/J", "conversion_reference"="DERIVED", "is_exact"=TRUE, "a"=0.0, "b"=1.0, "c"=3600000.0, "d"=0.0, "underlying_def"="", "description"=""}, {"symbol"="kg/MJ", "name"="kilogram per megajoule", "dimension"="T2/L2", "is_si_unit"=TRUE, "category"="derived", "base_unit"="kg/J", "conversion_reference"="DERIVED", "is_exact"=TRUE, "a"=0.0, "b"=1e-06, "c"=1.0, "d"=0.0, "underlying_def"="", "description"=""}, {"symbol"="lbm/(hp.h)", "name"="pound-mass per horsepower hour", "dimension"="T2/L2", "is_si_unit"=TRUE, "category"="derived", "base_unit"="kg/J", "conversion_reference"="DERIVED", "is_exact"=TRUE, "a"=0.0, "b"=0.45359237, "c"=2684519.537696173, "d"=0.0, "underlying_def"="", "description"=""}, {"symbol"="mg/J", "name"="milligram per joule", "dimension"="T2/L2", "is_si_unit"=TRUE, "category"="derived", "base_unit"="kg/J", "conversion_reference"="DERIVED", "is_exact"=TRUE, "a"=0.0, "b"=1e-06, "c"=1.0, "d"=0.0, "underlying_def"="", "description"=""}, {"symbol"="1/lbf", "name"="per pound-force", "dimension"="T2/LM", "is_si_unit"=TRUE, "category"="derived", "base_unit"="1/N", "conversion_reference"="DERIVED", "is_exact"=TRUE, "a"=0.0, "b"=1.0, "c"=4.4482216152605, "d"=0.0, "underlying_def"="", "description"=""}, {"symbol"="1/N", "name"="per Newton", "dimension"="T2/LM", "is_si_unit"=TRUE, "category"="derived", "base_unit"="", "conversion_reference"="", "is_exact"=FALSE, "a"=0.0, "b"=0.0, "c"=0.0, "d"=0.0, "underlying_def"="", "description"=""}, {"symbol"="B", "name"="bel", "dimension"="none", "is_si_unit"=TRUE, "category"="atom-allowed", "base_unit"="", "conversion_reference"="", "is_exact"=FALSE, "a"=0.0, "b"=0.0, "c"=0.0, "d"=0.0, "underlying_def"="", "description"="A unit of intensity. \n\t\t\t\tA bel is the base 10 logarithm of a power or amplitude ratio. \n\t\t\t\tIn using this unit it is important that the nature of the quantity be specified, and that any \n\t\t\t\treference value used be specified.\n\t\t\t"}, {"symbol"="dAPI", "name"="API gravity unit", "dimension"="none", "is_si_unit"=TRUE, "category"="atom-allowed", "base_unit"="", "conversion_reference"="", "is_exact"=FALSE, "a"=0.0, "b"=0.0, "c"=0.0, "d"=0.0, "underlying_def"="", "description"="A unit defined by the American Petroleum Institute for gravity of crude petroleum measurements. \n\t\t\t\tSee the API's Manual of Petroleum Measurement Standards (MPMS) chapter 9.1 and chapter 11.1 for \n\t\t\t\tinformation on this concept.\n\t\t\t"}, {"symbol"="gAPI", "name"="API gamma ray unit", "dimension"="none", "is_si_unit"=TRUE, "category"="atom-allowed", "base_unit"="", "conversion_reference"="", "is_exact"=FALSE, "a"=0.0, "b"=0.0, "c"=0.0, "d"=0.0, "underlying_def"="", "description"="A unit defined by the American Petroleum Institute for gamma ray log measurements."}, {"symbol"="nAPI", "name"="API neutron unit", "dimension"="none", "is_si_unit"=TRUE, "category"="atom-allowed", "base_unit"="", "conversion_reference"="", "is_exact"=FALSE, "a"=0.0, "b"=0.0, "c"=0.0, "d"=0.0, "underlying_def"="", "description"="A unit defined by the American Petroleum Institute for neutron log measurements."}, {"symbol"="O", "name"="octave", "dimension"="none", "is_si_unit"=TRUE, "category"="atom-allowed", "base_unit"="", "conversion_reference"="", "is_exact"=FALSE, "a"=0.0, "b"=0.0, "c"=0.0, "d"=0.0, "underlying_def"="", "description"="The number of octaves between two positive values is the base two logarithm of their ratio."}, {"symbol"="dB.mW", "name"="decibel milliwatt", "dimension"="none", "is_si_unit"=TRUE, "category"="derived", "base_unit"="B.W", "conversion_reference"="DERIVED", "is_exact"=TRUE, "a"=0.0, "b"=0.0001, "c"=1.0, "d"=0.0, "underlying_def"="", "description"=""}, {"symbol"="dB.MW", "name"="decibel megawatt", "dimension"="none", "is_si_unit"=TRUE, "category"="derived", "base_unit"="B.W", "conversion_reference"="DERIVED", "is_exact"=TRUE, "a"=0.0, "b"=100000.0, "c"=1.0, "d"=0.0, "underlying_def"="", "description"=""}, {"symbol"="dB.W", "name"="decibel watt", "dimension"="none", "is_si_unit"=TRUE, "category"="derived", "base_unit"="B.W", "conversion_reference"="DERIVED", "is_exact"=TRUE, "a"=0.0, "b"=0.1, "c"=1.0, "d"=0.0, "underlying_def"="", "description"=""}, {"symbol"="dB/ft", "name"="decibel per foot", "dimension"="none", "is_si_unit"=TRUE, "category"="derived", "base_unit"="B/m", "conversion_reference"="DERIVED", "is_exact"=TRUE, "a"=0.0, "b"=0.1, "c"=0.3048, "d"=0.0, "underlying_def"="", "description"=""}, {"symbol"="dB/km", "name"="decibel per kilometre", "dimension"="none", "is_si_unit"=TRUE, "category"="derived", "base_unit"="B/m", "conversion_reference"="DERIVED", "is_exact"=TRUE, "a"=0.0, "b"=0.0001, "c"=1.0, "d"=0.0, "underlying_def"="", "description"=""}, {"symbol"="dB/m", "name"="decibel per metre", "dimension"="none", "is_si_unit"=TRUE, "category"="derived", "base_unit"="B/m", "conversion_reference"="DERIVED", "is_exact"=TRUE, "a"=0.0, "b"=0.1, "c"=1.0, "d"=0.0, "underlying_def"="", "description"=""}, {"symbol"="dB/O", "name"="decibel per octave", "dimension"="none", "is_si_unit"=TRUE, "category"="derived", "base_unit"="B/O", "conversion_reference"="DERIVED", "is_exact"=TRUE, "a"=0.0, "b"=0.1, "c"=1.0, "d"=0.0, "underlying_def"="", "description"=""}, {"symbol"="B.W", "name"="bel watt", "dimension"="none", "is_si_unit"=TRUE, "category"="derived", "base_unit"="", "conversion_reference"="", "is_exact"=FALSE, "a"=0.0, "b"=0.0, "c"=0.0, "d"=0.0, "underlying_def"="", "description"=""}, {"symbol"="B/m", "name"="bel per metre", "dimension"="none", "is_si_unit"=TRUE, "category"="derived", "base_unit"="", "conversion_reference"="", "is_exact"=FALSE, "a"=0.0, "b"=0.0, "c"=0.0, "d"=0.0, "underlying_def"="", "description"=""}, {"symbol"="B/O", "name"="bel per octave", "dimension"="none", "is_si_unit"=TRUE, "category"="derived", "base_unit"="", "conversion_reference"="", "is_exact"=FALSE, "a"=0.0, "b"=0.0, "c"=0.0, "d"=0.0, "underlying_def"="", "description"="The power or amplitude variation that occurs over a doubling of the domain variable."}, {"symbol"="V/B", "name"="volt per bel", "dimension"="none", "is_si_unit"=TRUE, "category"="derived", "base_unit"="", "conversion_reference"="", "is_exact"=FALSE, "a"=0.0, "b"=0.0, "c"=0.0, "d"=0.0, "underlying_def"="", "description"=""}, {"symbol"="V/dB", "name"="volt per decibel", "dimension"="none", "is_si_unit"=TRUE, "category"="derived", "base_unit"="V/B", "conversion_reference"="DERIVED", "is_exact"=TRUE, "a"=0.0, "b"=10.0, "c"=1.0, "d"=0.0, "underlying_def"="", "description"=""}, {"symbol"="dB", "name"="decibel", "dimension"="none", "is_si_unit"=TRUE, "category"="prefixed", "base_unit"="B", "conversion_reference"="DERIVED", "is_exact"=TRUE, "a"=0.0, "b"=0.1, "c"=1.0, "d"=0.0, "underlying_def"="", "description"=""}]
  out "value out":dbl
  in  "value in":dbl
  in  "from_unit":string="m"
  in  "to_unit":string="in"
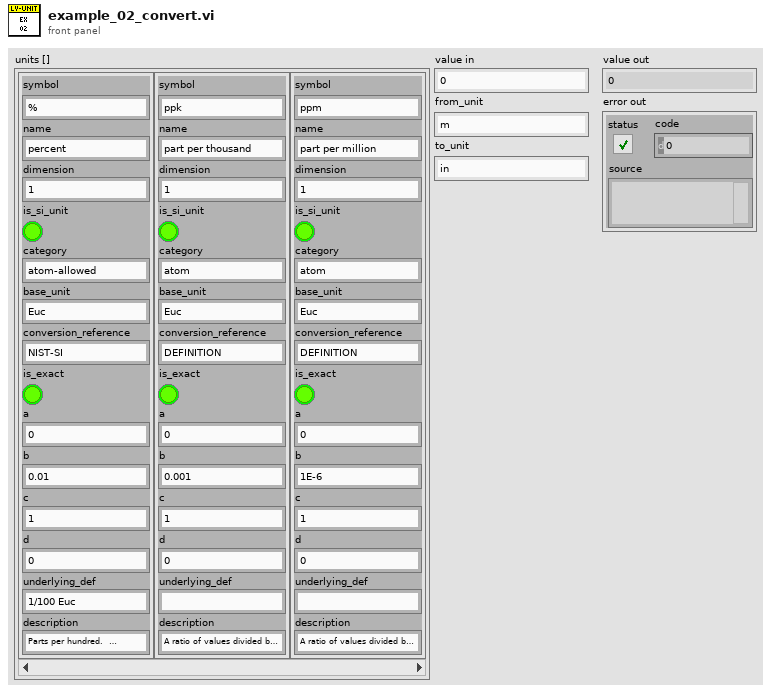
[diagram p1: front panel]
types:
  T1 = typedef "lv-unit-conversion.lvlib/unit.ctl" = cluster{"symbol":string, "name":string, "dimension":string, "is_si_unit":bool, "category":string, "base_unit":string, "conversion_reference":string, "is_exact":bool, "a":dbl, "b":dbl, "c":dbl, "d":dbl, "underlying_def":string, "description":string}
